vi "lawofsineangleb.vi"(9 "b":dbl format="%#_13g", 10 "Angle A":dbl format="%#_13g", 11 "a":dbl format="%#_13g") -> (3 "Angle B":dbl format="%#_13g")   [LabVIEW 2018]
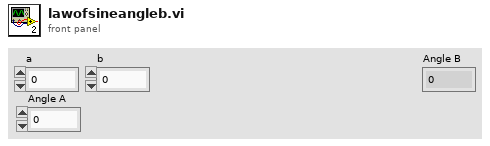
[diagram p1: front panel]
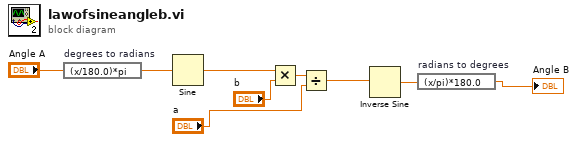
[diagram p0: block diagram]
diagram:
  n1 = expression code="(x/180.0)*pi" "degrees to radians"("Angle A") -> (w8:dbl)
  n2 = Sine(x=w8) -> (sin(x)=w7:dbl)
  n3 = Multiply(x=w7, y="b") -> (x*y=w4:dbl)
  n4 = Divide(x=w4, y="a") -> (x/y=w3:dbl)
  n5 = Inverse Sine(1:w3) -> (0:w2:dbl)
  n6 = expression code="(x/pi)*180.0" "radians to degrees"(w2) -> (→"Angle B":dbl)
